vi "Xeryon filter commands.vi"(3 "Letter in":string, 4 "Commands in":string[](array[string])) -> (1 "Commands out":string[](array[string]))   [LabVIEW 2019]
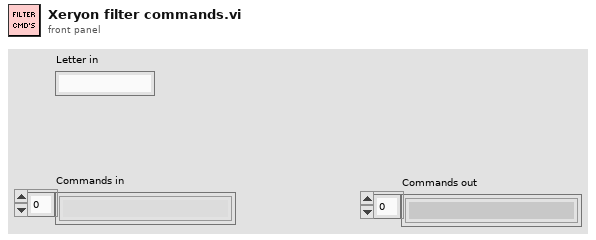
[diagram p1: front panel]
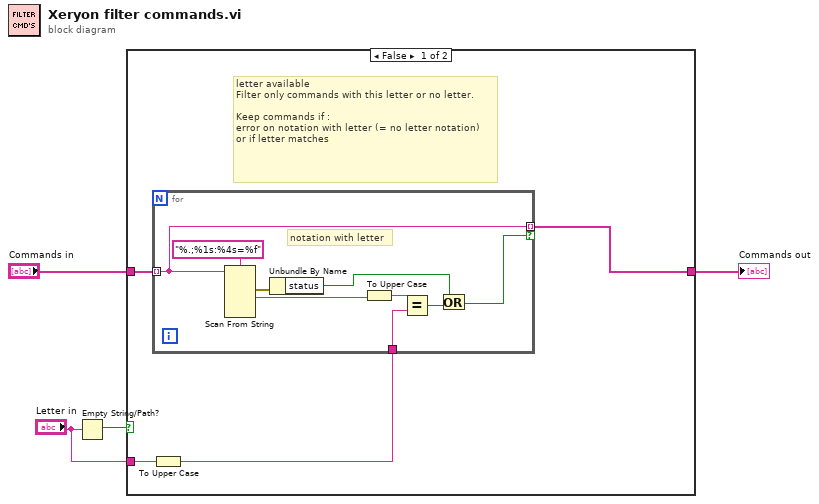
[diagram p0: block diagram]
diagram:
  n1 = Empty String/Path?(string/path="Letter in") -> (empty?=w4:bool)
  n2 = case shown="False" w4 {
    tunnel: [w5 w18] -> w2
    tunnel: "Commands in" -> [w8 w18]
    tunnel: "Letter in" -> [w7 _]
    frame False {
      # "letter available\nFilter only commands with this letter or no letter.\n\nKeep commands if :\nerror on notation with letter (= no letter notation)\nor if letter matches"
      n3 = To Upper Case(1:w7) -> (0:w6:string)
      n4 = for {
        tunnel: w8 -> [w10] mode=indexing
        tunnel: w6 -> [w13]
        tunnel: [w10] -> w5 mode=indexing if=w9
        # "notation with letter"
        n5 = Scan From String(format string="%.;%1s:%4s=%f", input string=w10) -> (error out=w16:errorcluster, output 1=w15:string)  [unwired: 7 in, 2 out]
        n6 = Unbundle By Name(w16) -> ("status"=w12:bool)
        n7 = To Upper Case(1:w15) -> (0:w14:string)
        n8 = Equal?(x=w14, y=w13) -> (x = y?=w11:bool)
        n9 = Or(x=w12, y=w11) -> (x .or. y?=w9:bool)
      }
    }
    frame True {
      # "empty - no letter\n\nSingle axis system"
    }
  }
  "Commands out" <- w2
